vi "Get Package Attributes.vi"(8 "error in":errorcluster, 10 "version":string, 11 "package name":string) -> (0 "error out":errorcluster, 1 "found?":bool, 2 "package attributes":T1={"Package Name"="", "Display name"="", "Version"="", "Display version"="", "Synopsis"="", "Description"="", "Maintainer"="", "Maintainer email address"="", "Category"="", "Homepage"="", "Release notes"="", "Depends"=[], "Recommends"=[], "Suggests"=[], "Conflicts"=[], "Provides"=[], "Replaces"=[], "Supplements"=[], "Enhances"=[], "Product"=FALSE, "User visible"=FALSE, "Installed size (KB)"=0, "Package filesize (bytes)"=0, "Architecture"="", "Agent"="file", "MD5Checksum"=""}, 3 "package name out":string)   [LabVIEW 2014, in "NIPM_API.lvlib"]
doc: "Returns the attributes for the specified version of a package"
uses:
  NIPM_API.lvlib
  _support/package attributes.ctl
panel:
  out "cmd standard output":string
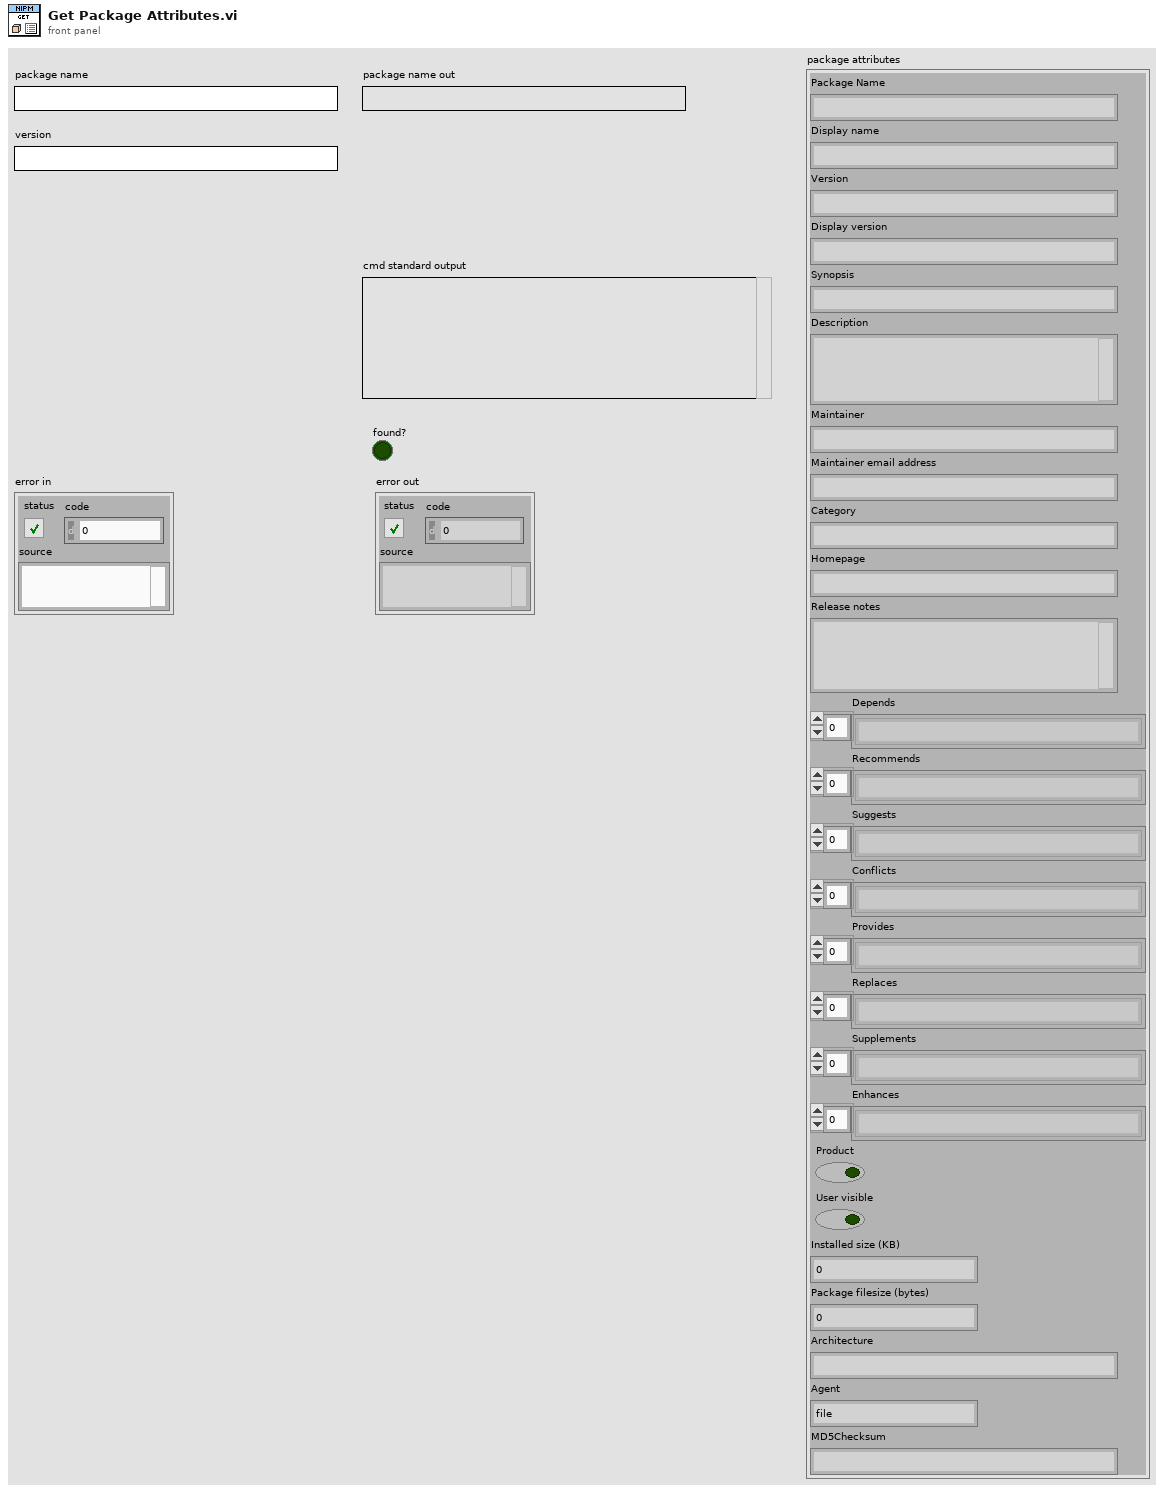
[diagram p1: front panel]
types:
  T1 = typedef "NIPM_API.lvlib/package attributes.ctl" = cluster{"Package Name":string, "Display name":string, "Version":string, "Display version":string, "Synopsis":string, "Description":string, "Maintainer":string, "Maintainer email address":string, "Category":string, "Homepage":string, "Release notes":string, "Depends":string[], "Recommends":string[], "Suggests":string[], "Conflicts":string[], "Provides":string[], "Replaces":string[], "Supplements":string[], "Enhances":string[], "Product":bool, "User visible":bool, "Installed size (KB)":u64, "Package filesize (bytes)":u64, "Architecture":string, "Agent":string, "MD5Checksum":string}
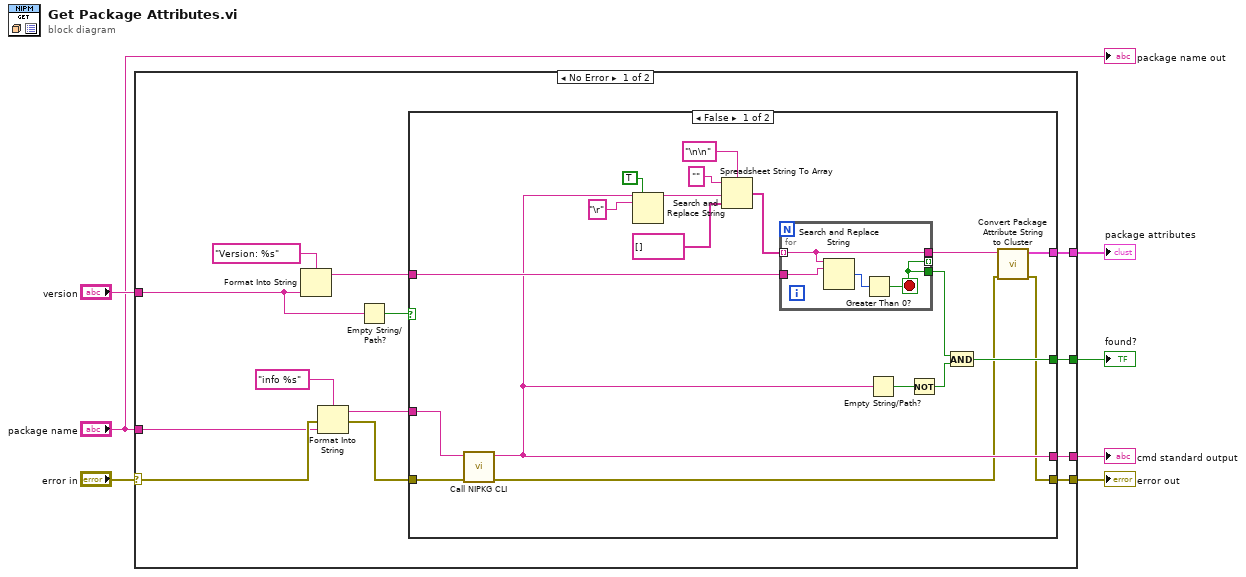
[diagram p0: block diagram]
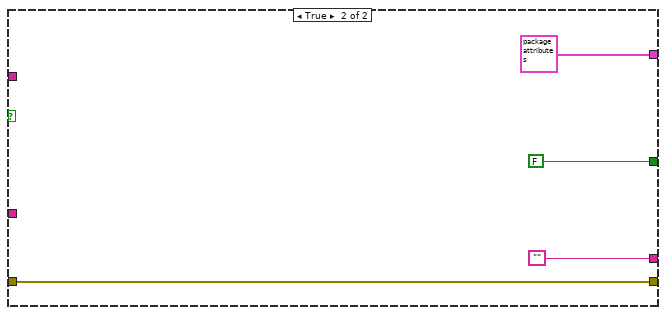
[diagram p2: hidden frame]
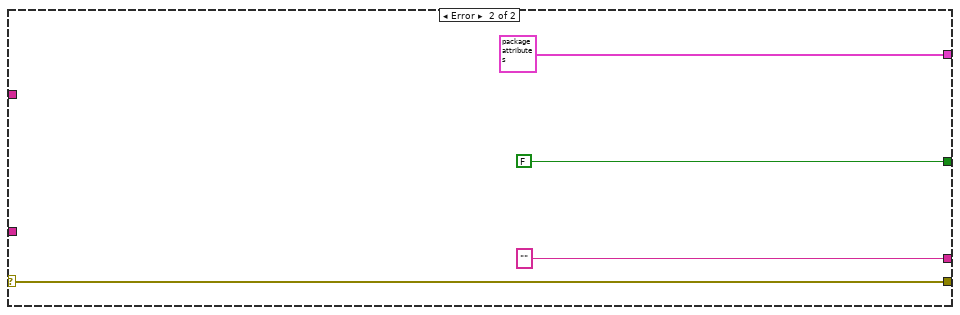
[diagram p3: hidden frame]
diagram:
  n1 = case shown="No Error" "error in" {
    selector: "error in" -> [w19 w51]
    tunnel: [w17 w51] -> w6
    tunnel: [w13 T1 {"Package Name"="", "Display name"="", "Version"="", "Display version"="", "Synopsis"="", "Description"="", "Maintainer"="", "Maintainer email address"="", "Category"="", "Homepage"="", "Release notes"="", "Depends"=[], "Recommends"=[], "Suggests"=[], "Conflicts"=[], "Provides"=[], "Replaces"=[], "Supplements"=[], "Enhances"=[], "Product"=FALSE, "User visible"=FALSE, "Installed size (KB)"=0, "Package filesize (bytes)"=0, "Architecture"="", "Agent"="file", "MD5Checksum"=""} ("package attributes")] -> w3
    tunnel: [w12 "" ("standard output")] -> w5
    tunnel: [w11 FALSE] -> w4
    tunnel: "version" -> [w9 _]
    tunnel: "package name" -> [w8 _]
    frame No Error {
      n2 = Format Into String(format string="Version: %s", w9) -> (resulting string=w14:string)  [unwired: 2 in, 1 out]
      n3 = Format Into String(format string="info %s", error in=w19, w8) -> (resulting string=w16:string, error out=w18:errorcluster)  [unwired: 1 in]
      n4 = Empty String/Path?(string/path=w9) -> (empty?=w10:bool)
      n5 = case shown="False" w10 {
        tunnel: w18 -> [w26 w46]
        tunnel: [w21 w46] -> w17
        tunnel: w16 -> [w27 _]
        tunnel: w14 -> [w32 _]
        tunnel: [w23 T1 {"Package Name"="", "Display name"="", "Version"="", "Display version"="", "Synopsis"="", "Description"="", "Maintainer"="", "Maintainer email address"="", "Category"="", "Homepage"="", "Release notes"="", "Depends"=[], "Recommends"=[], "Suggests"=[], "Conflicts"=[], "Provides"=[], "Replaces"=[], "Supplements"=[], "Enhances"=[], "Product"=FALSE, "User visible"=FALSE, "Installed size (KB)"=0, "Package filesize (bytes)"=0, "Architecture"="", "Agent"="file", "MD5Checksum"=""} ("package attributes")] -> w13
        tunnel: [w25 ""] -> w12
        tunnel: [w31 FALSE] -> w11
        frame False {
          n6 = call "Call NIPKG CLI.vi"("error in (no error)"=w26, "command"=w27) -> ("error out"=w22:errorcluster, "command line standard output"=w25:string)  [unwired: 8 in]
          n7 = Search and Replace String(replace all?=TRUE ("replace all? (F)"), input string=w25, search string="\r") -> (result string=w37:string)  [unwired: 5 in, 3 out]
          n8 = Spreadsheet String To Array(delimiter (Tab)="\n\n", format string="", spreadsheet string=w37, array type (2D Dbl)=string[] []) -> (array=w33:string[])
          n9 = for {
            tunnel: w33 -> [w41] mode=indexing
            tunnel: w32 -> [w42]
            tunnel: [w41] -> w24 if=w43
            tunnel: [w43] -> _ mode=indexing
            tunnel: [w43] -> w28
            stop <- w43 stop-if-true
            n10 = Search and Replace String(input string=w41, search string=w42) -> (number of replacements=w40:i32)  [unwired: 6 in, 3 out]
            n11 = Greater Than 0?(x=w40) -> (x > 0?=w43:bool)
          }
          n12 = Empty String/Path?(string/path=w25) -> (empty?=w30:bool)
          n13 = Not(x=w30) -> (.not. x?=w29:bool)
          n14 = And(x=w28, y=w29) -> (x .and. y?=w31:bool)
          n15 = call "Convert Package Attribute String to Cluster.vi"("error in (no error)"=w22, "nipkg CLI info string"=w24) -> ("error out"=w21:errorcluster, "package attributes"=w23:T1)  [unwired: 8 in]
        }
        frame True {
        }
      }
    }
    frame Error {
    }
  }
  "error out" <- w6
  "cmd standard output" <- w5
  "found?" <- w4
  "package attributes" <- w3
  "package name out" <- "package name"
